vi "Test_IncrementValuePublication_String_ErrorReturned.vi"(8 "error in (no error)":errorcluster, 11 "TestCase in":refnum<class "TestPublicationPolicy.lvclass">) -> (0 "error out":errorcluster, 3 "TestCase out":refnum<class "TestPublicationPolicy.lvclass">)   [LabVIEW 2017, in "PublicationPolicy.lvlib" / "TestPublicationPolicy.lvclass"]
uses:
  TestPublicationPolicy.lvclass
  IncrementValuePublication/IncrementValuePublication.lvclass
  C:/Git/mva-framework/Framework/IMediator/IPublicationPolicy/IPublicationPolicy.lvclass
  IMediator/IPublicationPolicy/IPublicationPolicy.lvclass
  Transport/QueueTransport/QueueTransport.lvclass/QueueTransport.ctl
  IMediator/PublishRequest/PublishRequest.lvclass/PublishRequest.ctl
  IMediator/MutexedPublishRequest/MutexedPublishRequest.lvclass/MutexedPublishRequest.ctl
  IMediator/PublishRequest/Write Publish Request Data.vi
  Transport/QueueTransport/QueueTransport.lvclass
  C:/Git/mva-framework/Framework/IMediator/ITransport/ITransport.lvclass
  IMediator/MutexedPublishRequest/MutexedPublishRequest.lvclass
  C:/Git/mva-framework/Framework/IMediator/PublishRequest/PublishRequest.lvclass
  <vilib>/Utility/error.llb/Error Cluster From Error Code.vi
panel:
  out "Publish Return Error":errorcluster
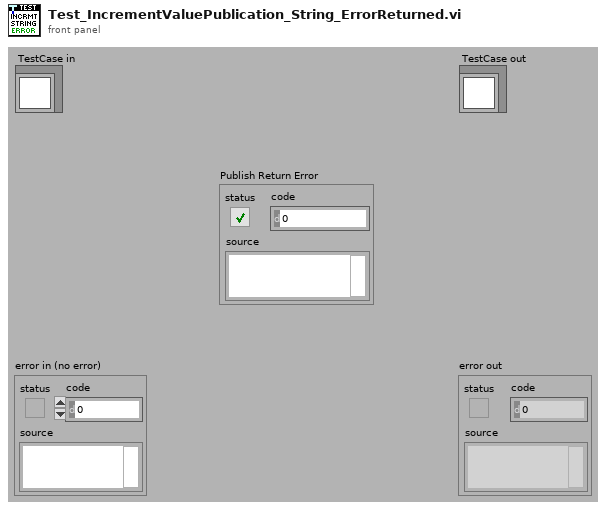
[diagram p1: front panel]
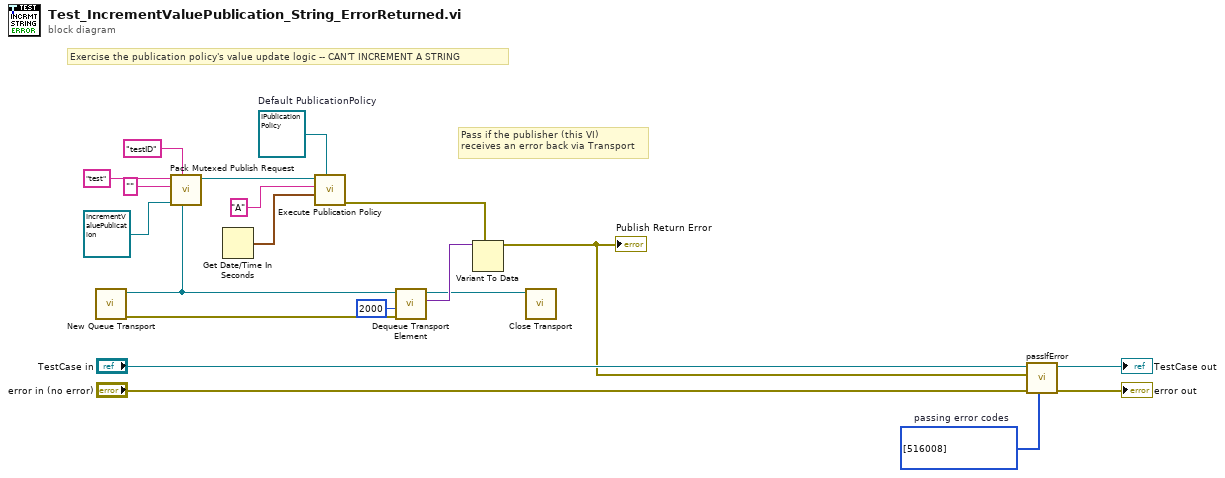
[diagram p0: block diagram]
diagram:
  w1 = i32[] [516008]  # passing error codes
  w12 = refnum<class "IPublicationPolicy.lvclass"> refnum  # Default PublicationPolicy
  # "Pass if the publisher (this VI)\nreceives an error back via Transport"
  # "Exercise the publication policy's value update logic -- CAN'T INCREMENT A STRING"
  n1 = call "New Queue Transport.vi"() -> ("error out"=w7:errorcluster, "QueueTransport"=w8:refnum<class "QueueTransport.lvclass">)  [unwired: 10 in]
  n2 = call "Pack Mutexed Publish Request.vi"("Return Error Transport"=w8, "Publisher ID"="testID", "PublicationPolicy"=refnum<class "IncrementValuePublication.lvclass"> refnum ("PublicationPolicy.lvlib:IncrementValuePublication.lvclass"), "Datum Value or Type"="" ("Data to Publish"), "Datum Name"="test") -> ("MutexedPublishRequest Out"=w14:refnum<class "MutexedPublishRequest.lvclass">)  [unwired: 6 in]
  n3 = Get Date/Time In Seconds() -> (seconds since 1Jan1904=w15:timestamp)
  n4 = call-dynamic "Execute Publication Policy.vi"("Default PublicationPolicy"=w12, "Last Publish Time"=w15, "Last Published Value"="A", "MutexedPublishRequest"=w14) -> ("error out (Reject Publication)"=w3:errorcluster)  [unwired: 5 in, 2 out]
  n5 = call "Dequeue Transport Element.vi"("error in (no error)"=w7, "Timeout In ms (-1)"=2000, "QueueTransport in"=w8) -> ("Data"=w5:variant, "QueueTransport out"=w4:refnum<class "QueueTransport.lvclass">)  [unwired: 5 in, 2 out]
  n6 = Variant To Data(type=w3, Variant=w5) -> (data=w2:errorcluster)  [unwired: 1 in, 1 out]
  "Publish Return Error" <- w2
  n7 = call-dynamic "Close Transport.vi"("QueueTransport in"=w4) -> ()  [unwired: 10 in, 1 out]
  n8 = call-dynamic "passIfError.vi"("passing error codes (default = any error code)"=w1, "error in (no error)"="error in (no error)", "error"=w2, "TestCase in"="TestCase in") -> ("error out"=→"error out":errorcluster, "TestCase out"=→"TestCase out":refnum<class "TestPublicationPolicy.lvclass">)  [unwired: 6 in]
